vi "Aeroprobe.vi"() -> (5 "Plug in titles":string[](array[string]), 7 "Plug in values":string[](array[string]))   [LabVIEW 2010]
uses:
  Globals/Meas_global.vi
panel:
  out "p-p(0)/mmH2O":dbl[](array[numeric])
  out "Temperature/C":dbl
  out "Pressure/mBar":dbl
  out "timeOfzero":timestamp
  out "zeroShift/mmH2O":dbl[](array[numeric])
  in  "Mode":enum32{"Measure", "Take Zeroes"}(radio)
  out "Velocity":dbl
  out "W":dbl
  out "V":dbl
  out "U":dbl
  # "!!  5-hole 1-5 must be connected to Channels 1-5   !!\n!! There must be a zeroth channel preceding them  !!"
  # "Zero Info"
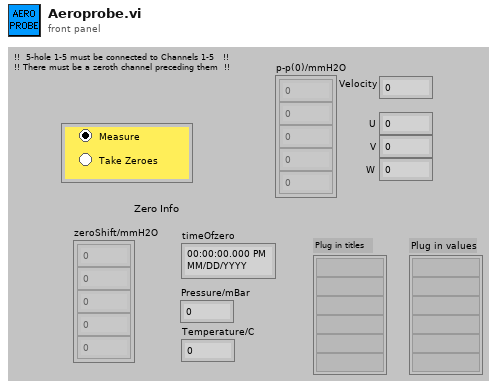
[diagram p1: front panel]
types:
  T1 = typedef "Velocity_cluster.ctl" = cluster{"Name":string, "U":dbl, "u^2":dbl, "u^3/(u^2)^(1.5)":dbl, "u^4/(u^2)^2 -3":dbl, "% u'/U":dbl, "Mean % Err":dbl, "u^4":dbl}
  T2 = cluster{"Velocity Cluster Array[0]":T1, "Velocity Cluster Array[1]":T1, "Velocity Cluster Array[2]":T1, "Velocity Cluster Array[3]":T1, "Velocity Cluster Array[4]":T1, "Velocity Cluster Array[5]":T1, "Velocity Cluster Array[6]":T1}
  T3 = cluster{"[0]":dbl, "[1]":dbl, "[2]":dbl, "[3]":dbl, "[4]":dbl}
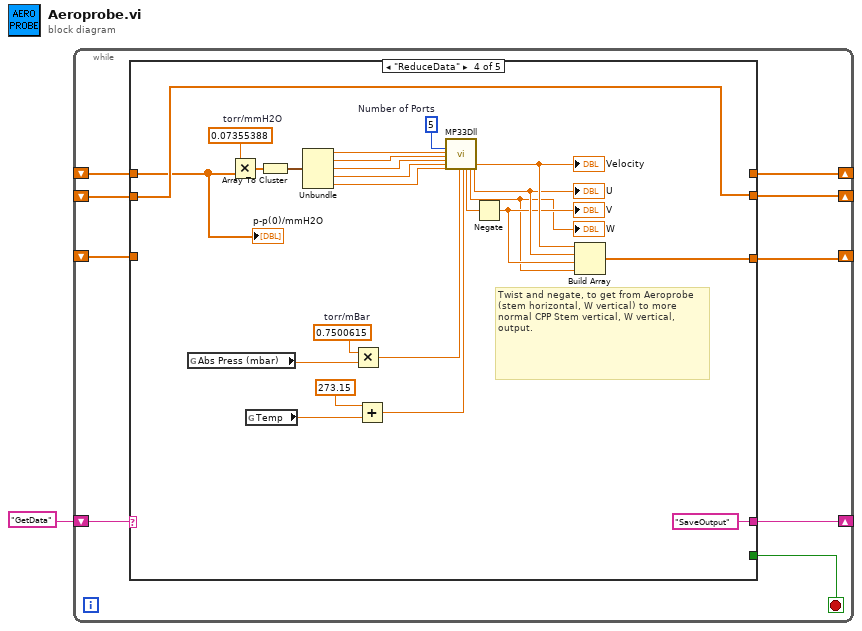
[diagram p0: block diagram]
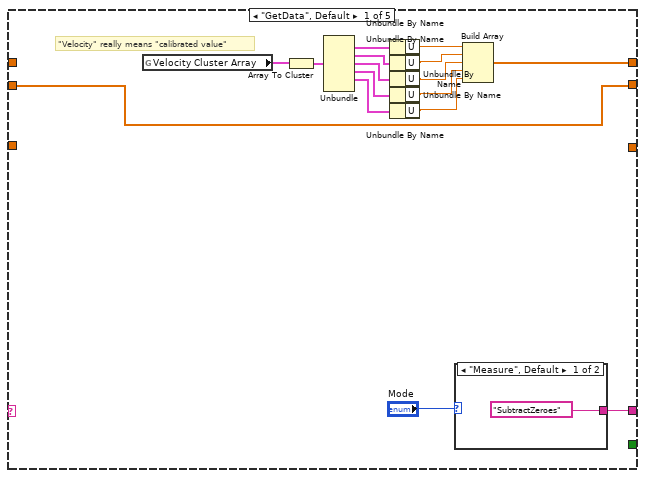
[diagram p2: hidden frame]
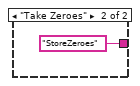
[diagram p3: hidden frame]
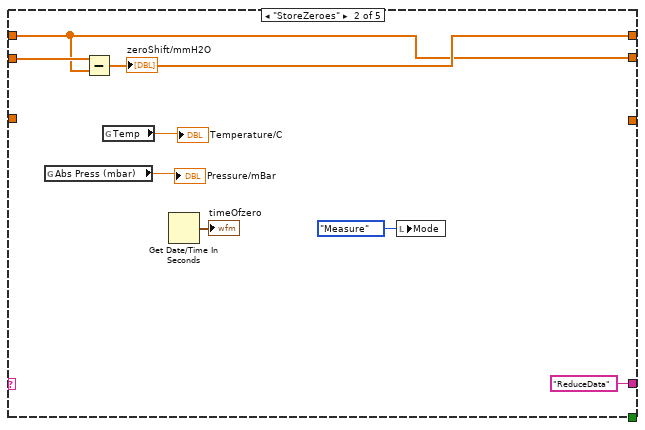
[diagram p4: hidden frame]
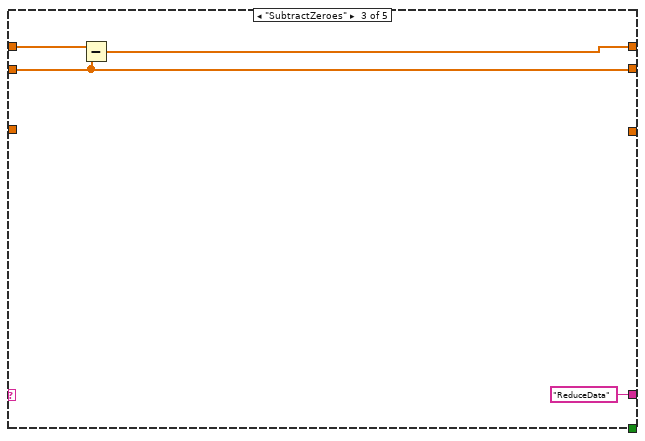
[diagram p5: hidden frame]
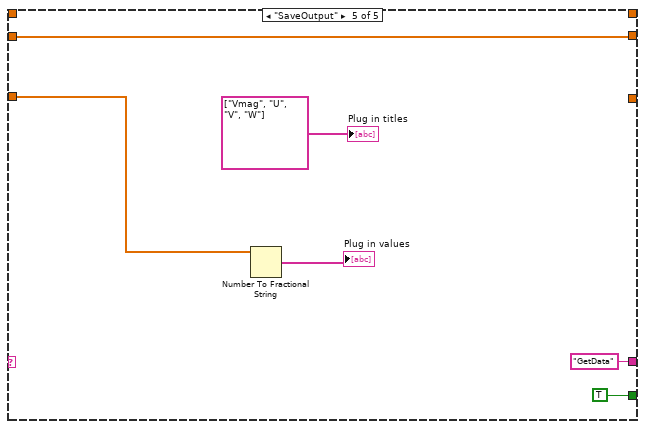
[diagram p6: hidden frame]
diagram:
  n1 = while {
    shift-right: [w9] -> _
    shift-left: "GetData" -> [w10]
    shift-right: [w8] -> _
    shift-left: _ -> [w6]
    shift-right: [w7] -> _
    shift-left: _ -> [w5]
    shift-right: [w4] -> _
    shift-left: _ -> [w3]
    stop <- w2 stop-if-true
    n2 = case shown="\"ReduceData\"" w10 {
      tunnel: [w19 "ReduceData" "ReduceData" "SaveOutput" "GetData"] -> w9
      tunnel: [w12 w34 w39 _ _] -> w8
      tunnel: [w11 w29 w38 w50 w70] -> w7
      tunnel: w6 -> [_ w29 w40 w41 _]
      tunnel: w5 -> [w11 w36 w38 w50 w70]
      tunnel: [_ _ _ w47 _] -> w4
      tunnel: w3 -> [_ _ _ _ w68]
      tunnel: [_ _ _ _ TRUE] -> w2
      frame "GetData", Default {
        # "\"Velocity\" really means \"calibrated value\""
        n3 = global read "Meas_global.vi" "Velocity Cluster Array"() -> (w20:T1[])
        n4 = Array To Cluster(array=w20) -> (cluster=w21:T2)
        n5 = Unbundle(w21) -> ("Velocity Cluster Array[1]"=w22:T1, "Velocity Cluster Array[2]"=w23:T1, "Velocity Cluster Array[3]"=w24:T1, "Velocity Cluster Array[4]"=w25:T1, "Velocity Cluster Array[5]"=w26:T1)  [unwired: 2 out]
        n6 = Unbundle By Name(w22) -> ("U"=w17:dbl)
        n7 = Unbundle By Name(w23) -> ("U"=w16:dbl)
        n8 = Unbundle By Name(w24) -> ("U"=w15:dbl)
        n9 = Unbundle By Name(w25) -> ("U"=w14:dbl)
        n10 = Unbundle By Name(w26) -> ("U"=w13:dbl)
        n11 = case shown="\"Measure\", Default" "Mode" {
          tunnel: ["SubtractZeroes" "StoreZeroes"] -> w19
          frame "Measure", Default {
          }
          frame "Take Zeroes" {
          }
        }
        n12 = Build Array(w17, w16, w15, w14, w13) -> (w12:dbl[])
      }
      frame "StoreZeroes" {
        n13 = global read "Meas_global.vi" "Abs Press (mbar)"() -> (→"Pressure/mBar":dbl)
        n14 = Subtract(x=w36, y=w29) -> (x-y=w34:dbl[])
        "zeroShift/mmH2O" <- w34
        n15 = global read "Meas_global.vi" "Temp"() -> (→"Temperature/C":dbl)
        n16 = Get Date/Time In Seconds() -> (seconds since 1Jan1904=→"timeOfzero":timestamp)
        n17 = local write "Mode"(enum32{"Measure", "Take Zeroes"}."Measure" ("Mode")) -> ()
      }
      frame "SubtractZeroes" {
        n18 = Subtract(x=w40, y=w38) -> (x-y=w39:dbl[])
      }
      frame "ReduceData" {
        w59 = 0.07355388  # torr/mmH2O
        w63 = 0.7500615  # torr/mBar
        w60 = 5  # Number of Ports
        # "Twist and negate, to get from Aeroprobe (stem horizontal, W vertical) to more normal CPP Stem vertical, W vertical, output."
        n19 = global read "Meas_global.vi" "Abs Press (mbar)"() -> (w45:dbl)
        n20 = Multiply(x=w59, y=w41) -> (x*y=w58:dbl[])
        n21 = global read "Meas_global.vi" "Temp"() -> (w46:dbl)
        n22 = Array To Cluster(array=w58) -> (cluster=w57:T3)
        n23 = Unbundle(w57) -> ("[0]"=w56:dbl, "[1]"=w55:dbl, "[2]"=w54:dbl, "[3]"=w53:dbl, "[4]"=w52:dbl)
        n24 = Multiply(x=w63, y=w45) -> (x*y=w62:dbl)
        n25 = Add(x=273.15, y=w46) -> (x+y=w64:dbl)
        n26 = call "MP33Dll.vi"("Number of Ports"=w60, "P1 Torr"=w56, "P2 Torr"=w55, "P3 Torr"=w54, "P4 Torr"=w53, "P5 Torr"=w52, "Pref Torr"=w62, "TTot Kelvin"=w64) -> ("w m/s"=w44:dbl, "v m/s"=w42:dbl, "VMagn m/s"=w49:dbl, "u  m/s"=w48:dbl)  [unwired: 10 in, 6 out]
        "U" <- w48
        "W" <- w42
        "Velocity" <- w49
        n27 = Negate(x=w44) -> (-x=w43:dbl)
        "V" <- w43
        n28 = Build Array(w49, w48, w43, w42) -> (w47:dbl[])
        "p-p(0)/mmH2O" <- w41
      }
      frame "SaveOutput" {
        n29 = Number To Fractional String(number=w68) -> (F-format string=→"Plug in values":string[])  [unwired: 3 in]
        "Plug in titles" <- string[] ["Vmag", "U", "V", "W"] ("Plug in titles")
      }
    }
  }
